vi "Plot SJ Datafile.vi"() -> ()   [LabVIEW 2011]
uses:
  <vilib>/Utility/file.llb/Read From Spreadsheet File (string).vi
  <vilib>/Utility/file.llb/Read From Spreadsheet File (DBL).vi
  <vilib>/Analysis/NI_AALBase.lvlib
panel:
  in  "Sort?":bool
  out "Selected Data SD":dbl format="%.2e"
  out "All Data SD":dbl format="%.2e"
  out "All Data":cluster{dbl[], dbl[]}[](graph)
  in  "Disc ID List":i32[](listbox)
  out "Selected Data":cluster{dbl[], dbl[]}[](graph)
  in  "File Path Control":path
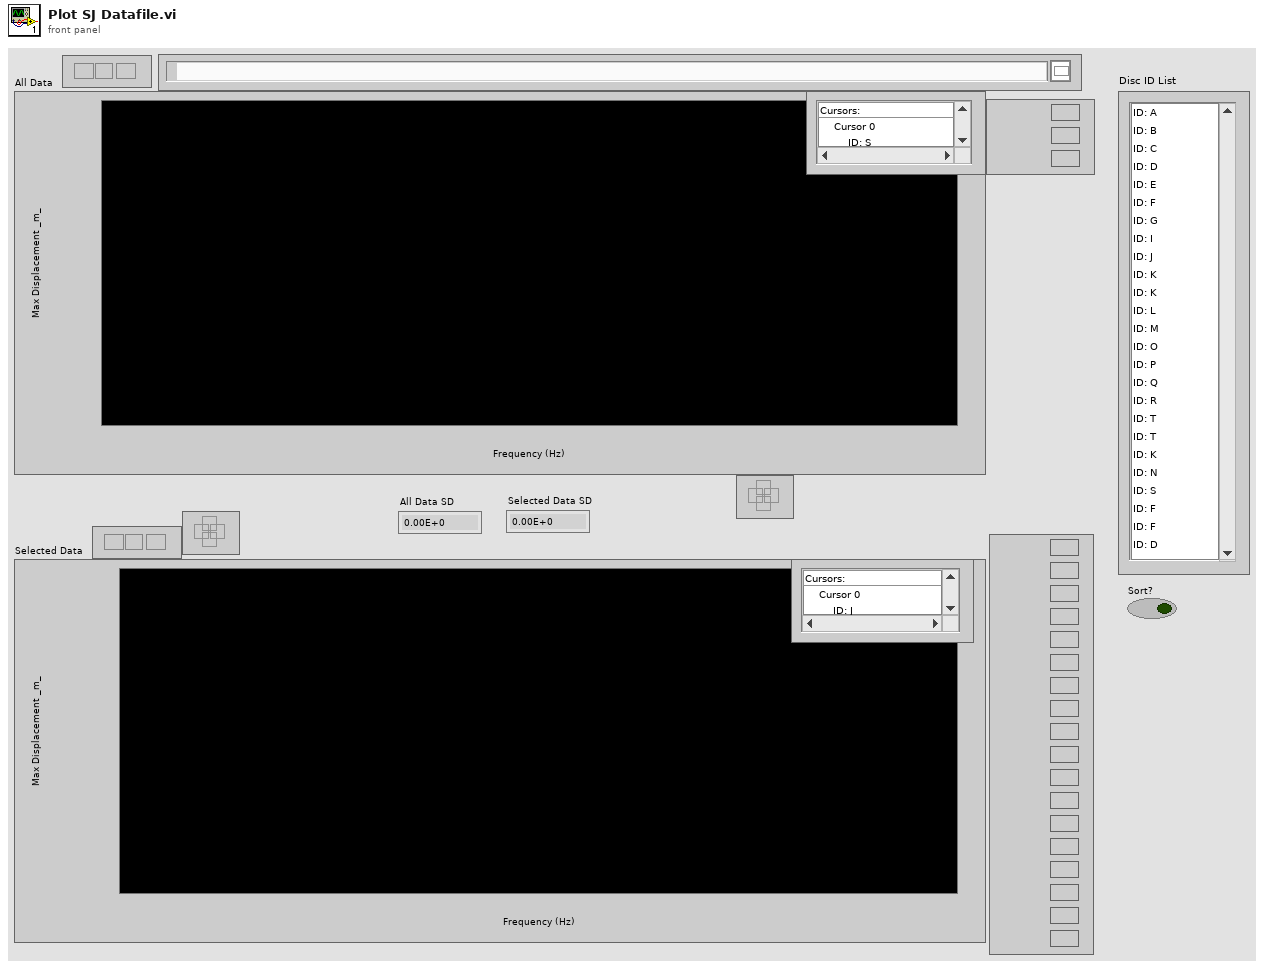
[diagram p1: front panel]
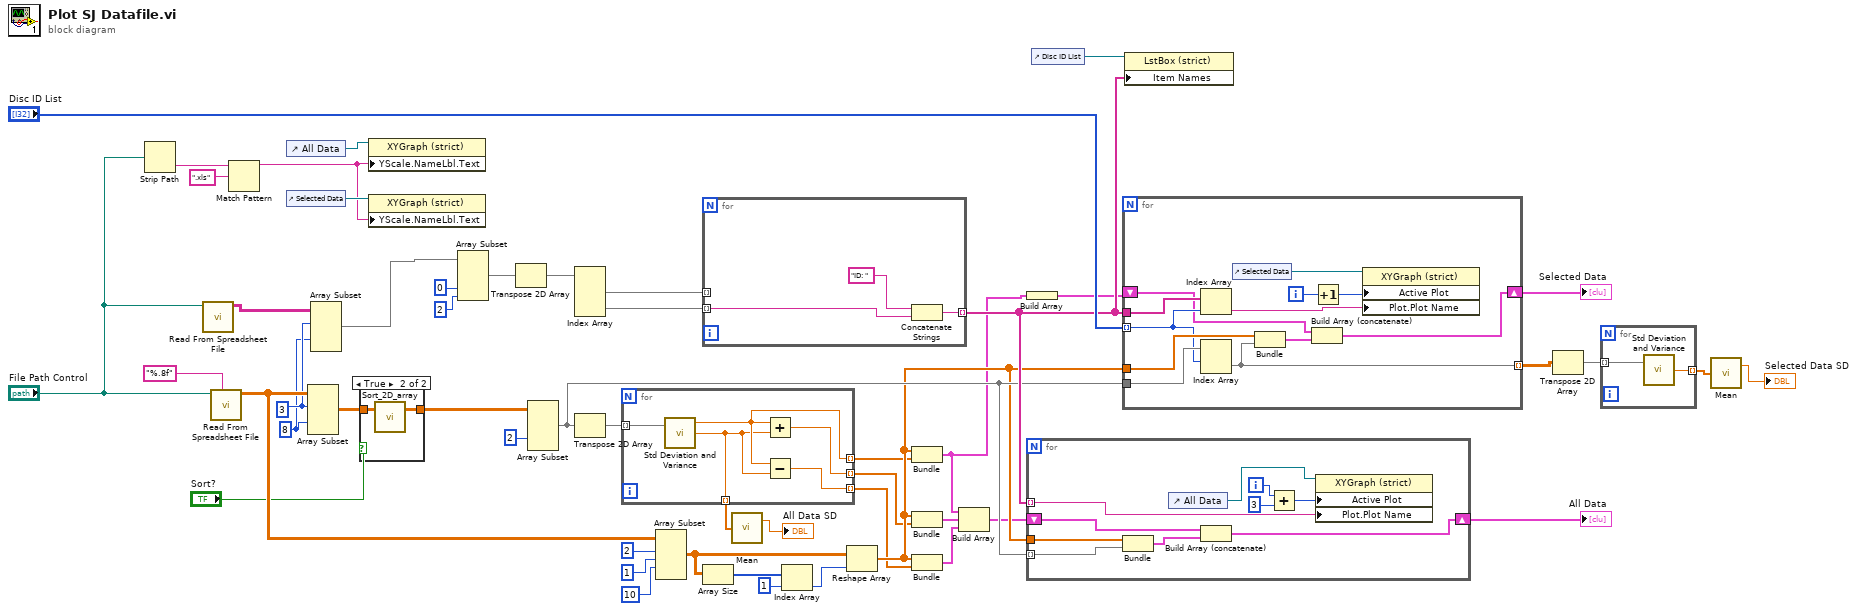
[diagram p0: block diagram]
diagram:
  w7 = 8 ("index")
  w8 = 3 ("index")
  n1 = Strip Path(path="File Path Control") -> (name=w31:string)  [unwired: 1 out]
  n2 = call-poly <vilib>:"Read From Spreadsheet File.vi"("file path (dialog if empty)"="File Path Control") -> ("all rows"=w6:string[][])  [unwired: 6 in, 4 out]
  n3 = call-poly <vilib>:"Read From Spreadsheet File.vi"("format (%.3f)"="%.8f", "file path (dialog if empty)"="File Path Control") -> ("all rows"=w43:dbl[][])  [unwired: 5 in, 4 out]
  n4 = Match Pattern(string=w31, regular expression=".xls") -> (before substring=w27:string)  [unwired: 1 in, 3 out]
  n5 = control-ref of="All Data"() -> (w29:refnum<vi>)
  n6 = control-ref of="Selected Data"() -> (w28:refnum<vi>)
  n7 = Array Subset(array=w43, index (row)=w8, index (col)=w7) -> (w41:dbl[][])  [unwired: 2 in]
  n8 = Array Subset(array=w6, index (row)=w8, index (col)=w7) -> (w4:string[][])  [unwired: 2 in]
  n9 = case shown="True" "Sort?" {
    tunnel: w41 -> [w52 w54]
    tunnel: [w52 w53] -> w3
    frame False {
    }
    frame True {
      n10 = call "Sort_2D_array.vi"("unsorted array"=w54) -> ("sorted array"=w53:dbl[][])  [unwired: 1 in, 1 out]
    }
  }
  n11 = property class="XYGraph (strict)"(reference=w29, "YScale.NameLbl.Text"=w27) -> ()  [unwired: 1 in, 2 out]
  n12 = property class="XYGraph (strict)"(reference=w28, "YScale.NameLbl.Text"=w27) -> ()  [unwired: 1 in, 2 out]
  n13 = Array Subset(array=w4, index (col)=0 ("index"), length (col)=2 ("length")) -> (w38:string[][])  [unwired: 2 in]
  n14 = Transpose 2D Array(2D array=w38) -> (transposed array=w42:string[][])
  n15 = Array Subset(array=w3, index (col)=2 ("index")) -> (w26:dbl[][])  [unwired: 3 in]
  n16 = Index Array(array=w42) -> (element #1=w2:string[], element #2=w1:string[])  [unwired: 4 in]
  n17 = Transpose 2D Array(2D array=w26) -> (transposed array=w25:dbl[][])
  n18 = for {
    tunnel: w25 -> [w59] mode=indexing
    tunnel: [w57] -> w23 mode=indexing
    tunnel: [w58] -> w22 mode=indexing
    tunnel: [w56] -> w21 mode=indexing
    tunnel: [w55] -> w17 mode=indexing
    n19 = call <vilib>:"Std Deviation and Variance.vi"("X"=w59) -> ("mean"=w57:dbl, "standard deviation"=w55:dbl)  [unwired: 1 in, 1 out]
    n20 = Add(x=w57, y=w55) -> (x+y=w58:dbl)
    n21 = Subtract(x=w57, y=w55) -> (x-y=w56:dbl)
  }
  n22 = Array Subset(array=w43, index (row)=2 ("index"), length (row)=1 ("length"), index (col)=10 ("index")) -> (w47:dbl[][])  [unwired: 1 in]
  n23 = for {
    tunnel: w1 -> [w60] mode=indexing
    tunnel: [w61] -> w33 mode=indexing
    tunnel: w2 -> [_] mode=indexing
    n24 = Concatenate Strings("ID: " ("string"), w60) -> (w61:string)
  }
  n25 = Array Size(array=w47) -> (size(s)=w46:i32[])
  n26 = call <vilib>:"Mean.vi"("X"=w17) -> ("mean"=→"All Data SD":dbl)  [unwired: 1 out]
  n27 = Index Array(array=w46, index=1) -> (element=w44:i32)
  n28 = Reshape Array(w47, w44) -> (w24:dbl[])
  n29 = Bundle(w24, w23) -> (w11:cluster{dbl[], dbl[]})  [unwired: 1 in]
  n30 = Bundle(w24, w22) -> (w20:cluster{dbl[], dbl[]})  [unwired: 1 in]
  n31 = Bundle(w24, w21) -> (w19:cluster{dbl[], dbl[]})  [unwired: 1 in]
  n32 = Build Array(w11, w20, w19) -> (w18:cluster{dbl[], dbl[]}[])
  n33 = Build Array(w11) -> (w10:cluster{dbl[], dbl[]}[])
  n34 = for {
    tunnel: w24 -> [w72]
    tunnel: w26 -> [w65] mode=indexing
    shift-right: [w69] -> w32
    shift-left: w18 -> [w68]
    tunnel: w33 -> [w67] mode=indexing
    i -> [w70]
    n35 = Bundle(w72, w65) -> (w71:cluster{dbl[], dbl[]})  [unwired: 1 in]
    n36 = control-ref of="All Data"() -> (w66:refnum<vi>)
    n37 = Build Array (concatenate)(w68, w71) -> (w69:cluster{dbl[], dbl[]}[])
    n38 = Add(x=w70, y=3) -> (x+y=w64:i32)
    n39 = property class="XYGraph (strict)"(reference=w66, "Active Plot"=w64, "Plot.Plot Name"=w67) -> ()  [unwired: 1 in, 2 out]
  }
  "All Data" <- w32
  n40 = control-ref of="Disc ID List"() -> (w36:refnum<vi>)
  n41 = for {
    tunnel: "Disc ID List" -> [w79] mode=indexing
    tunnel: w24 -> [w83]
    tunnel: w26 -> [w84]
    tunnel: w33 -> [w80]
    shift-right: [w77] -> w34
    shift-left: w10 -> [w76]
    tunnel: [w74] -> w14 mode=indexing
    i -> [w75]
    n42 = Index Array(array=w80, index=w79) -> (element=w78:string)
    n43 = Index Array(array=w84, index (row)=w79) -> (element=w74:dbl[])  [unwired: 1 in]
    n44 = control-ref of="Selected Data"() -> (w81:refnum<vi>)
    n45 = Bundle(w83, w74) -> (w82:cluster{dbl[], dbl[]})  [unwired: 1 in]
    n46 = Build Array (concatenate)(w76, w82) -> (w77:cluster{dbl[], dbl[]}[])
    n47 = Increment(x=w75) -> (x+1=w73:i32)
    n48 = property class="XYGraph (strict)"(reference=w81, "Active Plot"=w73, "Plot.Plot Name"=w78) -> ()  [unwired: 1 in, 2 out]
  }
  "Selected Data" <- w34
  n49 = property class="LstBox (strict)"(reference=w36, "Item Names"=w33) -> ()  [unwired: 1 in, 2 out]
  n50 = Transpose 2D Array(2D array=w14) -> (transposed array=w13:dbl[][])
  n51 = for {
    tunnel: w13 -> [w86] mode=indexing
    tunnel: [w85] -> w15 mode=indexing
    n52 = call <vilib>:"Std Deviation and Variance.vi"("X"=w86) -> ("standard deviation"=w85:dbl)  [unwired: 1 in, 2 out]
  }
  n53 = call <vilib>:"Mean.vi"("X"=w15) -> ("mean"=→"Selected Data SD":dbl)  [unwired: 1 out]
